vi "Steering Encoder Counter.vi"   [LabVIEW 2009]
uses:
  Motor Encoder Global.vi
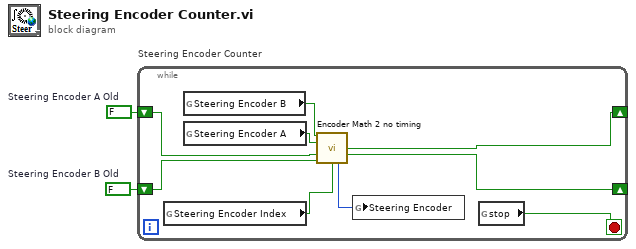
[diagram p0: block diagram]
diagram:
  w1 = FALSE  # Steering Encoder A Old
  w2 = FALSE  # Steering Encoder B Old
  n1 = while "Steering Encoder Counter" {
    shift-right: [w11] -> _
    shift-left: w1 -> [w10]
    shift-right: [w9] -> _
    shift-left: w2 -> [w8]
    stop <- w7 stop-if-true
    n2 = global read "Motor Encoder Global.vi" "Steering Encoder Index"() -> (w4:bool)
    n3 = global read "Motor Encoder Global.vi" "Steering Encoder B"() -> (w6:bool)
    n4 = global read "Motor Encoder Global.vi" "Steering Encoder A"() -> (w5:bool)
    n5 = call "Encoder Math 2 no timing.vi"("Encoder B"=w6, "Encoder A"=w5, "Encoder A Old"=w10, "Encoder B Old"=w8, "Encoder Index"=w4) -> ("Encoder A Old (sReg)"=w11:bool, "Encoder B Old (sReg)"=w9:bool, "Current count"=w3:i32)  [unwired: 5 in, 3 out]
    n6 = global write "Motor Encoder Global.vi" "Steering Encoder"(w3) -> ()
    n7 = global read "Motor Encoder Global.vi" "stop"() -> (w7:bool)
  }
